vi "FGV_Preis.vi"(7 "FGV-Status":T1, 8 "error in (no error)":errorcluster, 10 "Preis":dbl format="%#_13g") -> (0 "error out":errorcluster, 2 "Preis Output":dbl)   [LabVIEW 2023]
doc: "FGV-Preis"
uses:
  CONTROLS/fgv status.ctl
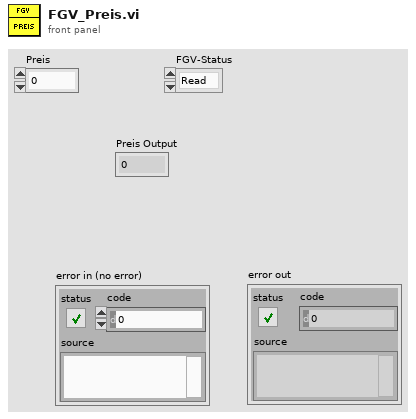
[diagram p1: front panel]
types:
  T1 = typedef "fgv status.ctl" = enum16{"Read", "Write"}
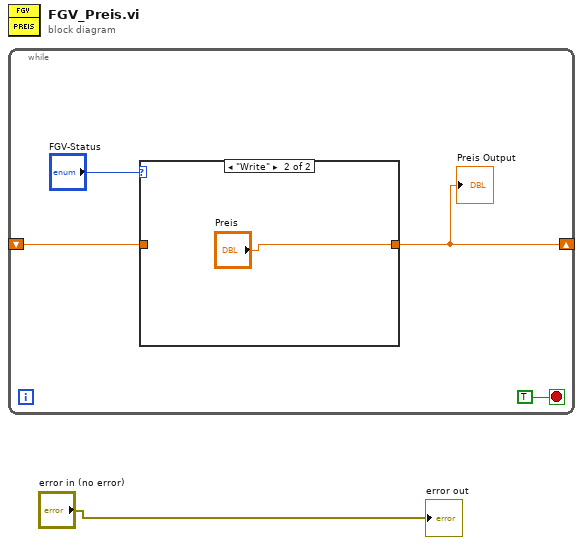
[diagram p0: block diagram]
diagram:
  n1 = while {
    shift-right: [w3] -> _
    shift-left: _ -> [w2]
    stop <- TRUE stop-if-true
    n2 = case shown="\"Write\"" "FGV-Status" {
      tunnel: [w6 "Preis"] -> w3
      tunnel: w2 -> [w6 _]
      frame "Read", Default {
      }
      frame "Write" {
      }
    }
    "Preis Output" <- w3
  }
  "error out" <- "error in (no error)"
